vi "Log_fillename_create.vi"(11 "start path":path=path "") -> (3 "Log filename":path caption="selected path", 5 "lof file name":string)   [LabVIEW 2012]
panel:
  out "refnum out":refnum<file>
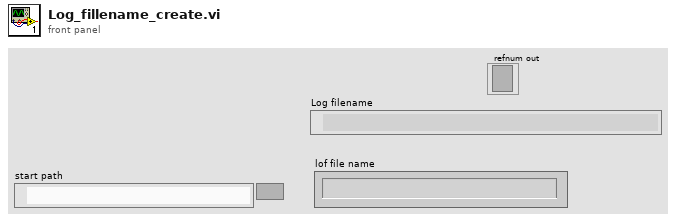
[diagram p1: front panel]
types:
  T1 = enum16{"open", "replace", "create", "open or create", "replace or create", "replace or create with confirmation"}
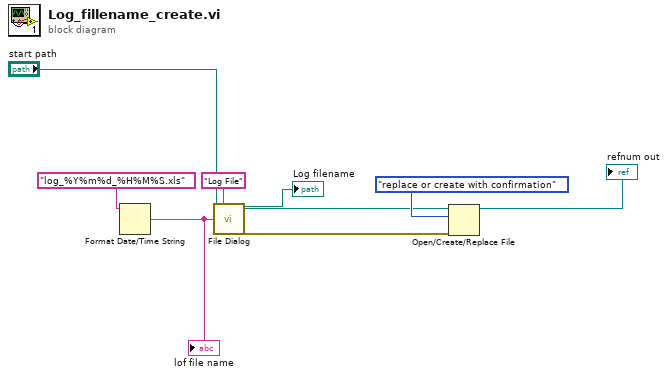
[diagram p0: block diagram]
diagram:
  n1 = Format Date/Time String(time format string (%c)="log_%Y%m%d_%H%M%S.xls" ("string")) -> (date/time string=w7:string)  [unwired: 2 out]
  "lof file name" <- w7
  n2 = call "File Dialog"("start path"="start path", "prompt"="Log File", "default name"=w7) -> ("selected path"=w5:path, "error out"=w3:errorcluster)  [unwired: 4 in, 7 out]
  "Log filename" <- w5
  n3 = Open/Create/Replace File(file path (use dialog)=w5, error in=w3, operation (0:open)=T1."replace or create with confirmation") -> (refnum out=→"refnum out":refnum<file>)  [unwired: 5 out]
